vi "SigSyn-Set Property.vi"(0 "StimChan In":T1 caption="Stimulus" {"Filter"."Stages"."IIR Filter"."Forward Coefficients" format="%.4f"; "Filter"."Stages"."IIR Filter"."Reverse Coefficients" format="%.4f"}, 7 "Property":string, 9 "Value":dbl) -> (4 "StimChan Out":T1={"Waveform"={"Type"=enum."Tone", "Tone"={"Frequency (kHz)"=0.0, "Last Freq"=0.0, "Last Phase"=0.0}, "Pulse Train"={"Pulse width (us)"=0.0, "Pulse rate (Hz)"=0.0, "Gap (ms)"=0.0, "Polarity"=enum."POS", "PT State"={"Template"=[], "Nperiod"=0, "Index"=0, "Pulse Rate (Hz)"=0.0, "Phase (cycles)"=0.0, "Noff"=0}, "Asynch"=FALSE}, "Noise"={"InvFilt"=FALSE, "Noise"=[], "CurPt"=0, "Aweight"=FALSE, "Seed"=0, "afile"=path ""}, "File"={"Filename"=path "", "Signal"=[], "Channel"=0, "stream"=FALSE, "offset"=0, "nreps"=0, "loops"=0}, "FMSweep"={"Rate (oct/s)"=0.0, "Fmin (Hz)"=0.0, "Fmax (Hz)"=0.0, "Ramp (ms)"=0.0, "Linear"=FALSE}, "Chirp Train"={"Params"={"Fmin (kHz)"=4.0, "Fmax (kHz)"=64.0, "Compensate"=FALSE, "Duration (ms)"=2.0}, "Data"={"WF"=[]}}, "Complex Tone"={"Params"={"F0 (Hz)"=0.0, "Band"={"Flow (Hz)"=0.0, "Fhigh (Hz)"=0.0}, "Phase"=enum."Cosine", "Min F0 (Hz)"=0.0, "Max F0 (Hz)"=0.0, "ContinRandPhase"=FALSE, "Max peak factor"=inf, "Max mod depth"=2.0, "MinHarmNum"=0, "MaxHarmNum"=0, "Level Mode"=enum."per component", "% jitter"=0.0}, "Data"={"Ncomp"=0, "MinHarm"=0, "Phase"=[], "Amplitude"=[], "Npts/frame"=0, "Last F0"=0.0, "Fmin"=0.0, "Fmax"=0.0, "Lslope"=0.0, "randphase"=FALSE, "overall rms"=FALSE, "fmult"=[], "jittered"=FALSE}}, "Moving Ripple"={"Params"={"Fmin"=0.0, "Fmax"=0.0, "Density"=0.0, "Velocity"=0.0, "Depth"=0.0, "Phase"=0.0, "Comp/oct"=0}, "Data"={"Freq"=[], "A"=[], "phase"=[], "Phase"=0.0}}}, "Filter"={"Type"=enum."Lowpass", "CF (kHz)"=0.0, "BW (kHz)"=0.0, "Cascade"=FALSE, "Quadrature"=FALSE, "Scale Factor"=0.0, "Stages"=[], "Class"=enum."Elliptic", "Order"=0, "BWUnits"=enum."Linear"}, "Burst"={"Active"=FALSE, "Delay (ms)"=0.0, "Duration (ms)"=0.0, "Ramp (ms)"=0.0, "Rate (Hz)"=0.0, "Trepeat (ms)"=0.0, "Repeat"=FALSE}, "Level"={"Level"=0.0, "Units"=enum."dB atten", "Max"=0.0, "Multiplier"=0.0, "Cal File"=path "", "Cal"={"Freq (Hz)"=[], "Mag (dB SPL)"=[], "Phase (deg)"=[]}}, "Name"="", "Advanced"={"Rep Mask"="", "AltPol"=FALSE, "Var"="", "Expr"="", "Persist"=FALSE}, "SAM"={"Active"=FALSE, "Frequency (Hz)"=0.0, "Depth"=0.0, "Init Phase (cycles)"=0.0, "phase (degrees)"=0.0, "Asynch"=FALSE}} {"Filter"."Stages"."IIR Filter"."Forward Coefficients" format="%.4f"; "Filter"."Stages"."IIR Filter"."Reverse Coefficients" format="%.4f"})   [LabVIEW 2015]
uses:
  Controls/Stimulus Channel (Full)/Full Stimulus Channel Data.ctl
  Controls/Waveform XCtl/Waveform Data.ctl
  Controls/Waveform XCtl/Waveform Enum.ctl
  Waveform VIs/Tone VIs/Tone Params.ctl
  Waveform VIs/Pulse Train VIs/Pulse Train Params.ctl
  Waveform VIs/Pulse Train VIs/Pulse Polarity.ctl
  Waveform VIs/Pulse Train VIs/PT-Continuous State.ctl
  Waveform VIs/Noise VIs/Noise Params.ctl
  Waveform VIs/File VIs/StimFile-Params.ctl
  Waveform VIs/FM Sweep VIs/FM Sweep Params.ctl
  Waveform VIs/Chirp Train VIs/Chirp Train.ctl
  Waveform VIs/Chirp Train VIs/Chirp Train Params.ctl
  Waveform VIs/Complex Tone VIs/CT-Params.ctl
  Waveform VIs/Complex Tone VIs/CT-Phase Enum.ctl
  Waveform VIs/Complex Tone VIs/CT-Runtime Data.ctl
  Waveform VIs/Moving Ripple VIs/Moving Ripple.ctl
  Waveform VIs/Moving Ripple VIs/Moving Ripple.Params.ctl
  Waveform VIs/Moving Ripple VIs/Moving Ripple.Data.ctl
  Controls/Advanced Filter XCtl/Filter Data.ctl
  Filter VIs/Filter-Bandwidth Units.ctl
  Controls/Burst XCtl/Burst Data.ctl
  Controls/Level XCtl/Level Data.ctl
  Controls/Level XCtl/Level Units.ctl
  Controls/Advanced Options XCtl/Advanced Stimulus Options.ctl
  Modulation VIs/SAM VIs/SAM Params.ctl
  <vilib>/regexp/Match Regular Expression.xnode
  Controls/Advanced Filter XCtl/Advanced Filter XCtl.xctl
  Controls/Level XCtl/Level XCtl.xctl
  Controls/Burst XCtl/Burst Control.xctl
  Controls/Waveform XCtl/Waveform XCtl.xctl
  Controls/Advanced Options XCtl/Advanced Stimulus Options.xctl
  Controls/Stimulus Channel (Full)/Stimulus Channel (Full).xctl
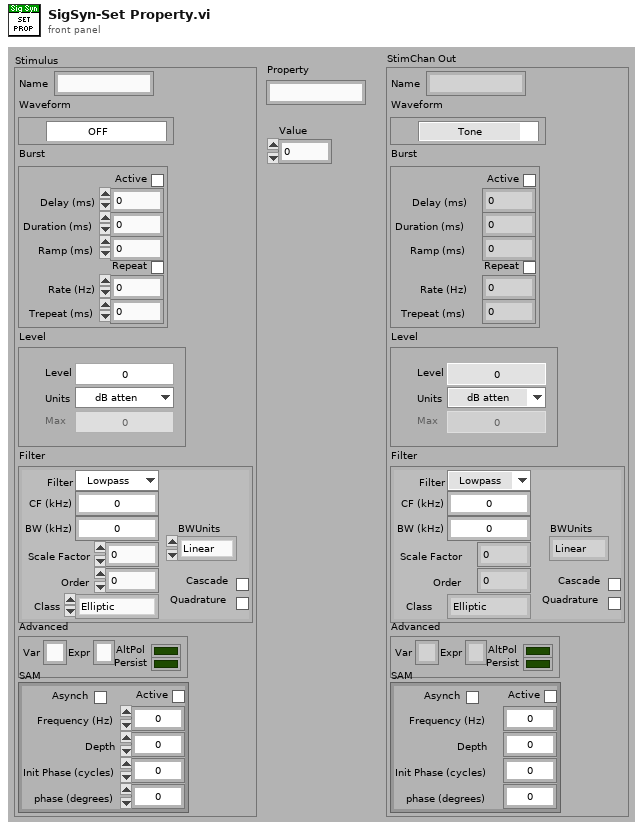
[diagram p1: front panel]
types:
  T1 = typedef "Stimulus Channel (Full).xctl/Full Stimulus Channel Data.ctl" = cluster{"Waveform":T2, "Filter":T19, "Burst":T21, "Level":T22, "Name":string, "Advanced":T24, "SAM":T25}
  T2 = typedef "Waveform XCtl.xctl/Waveform Data.ctl" = cluster{"Type":T3, "Tone":T4, "Pulse Train":T5, "Noise":T8, "File":T9, "FMSweep":T10, "Chirp Train":T11, "Complex Tone":cluster{"Params":T13, "Data":T15}, "Moving Ripple":T16}
  T3 = typedef "Waveform Enum.ctl" = enum16{"OFF", "Tone", "Noise", "Pulse Train", "File", "FM Sweep", "Chirp Train", "Complex Tone", "FM Tone", "Moving Ripple"}
  T4 = typedef "Tone Params.ctl" = cluster{"Frequency (kHz)":dbl, "Last Freq":dbl, "Last Phase":dbl}
  T5 = typedef "Pulse Train Params.ctl" = cluster{"Pulse width (us)":dbl, "Pulse rate (Hz)":dbl, "Gap (ms)":dbl, "Polarity":T6, "PT State":T7, "Asynch":bool}
  T6 = typedef "Pulse Polarity.ctl" = enum16{"POS", "NEG", "POS-NEG", "NEG-POS"}
  T7 = typedef "PT-Continuous State.ctl" = cluster{"Template":dbl[], "Nperiod":i32, "Index":i32, "Pulse Rate (Hz)":dbl, "Phase (cycles)":dbl, "Noff":i32}
  T8 = typedef "Noise Params.ctl" = cluster{"InvFilt":bool, "Noise":dbl[], "CurPt":i32, "Aweight":bool, "Seed":i32, "afile":path}
  T9 = typedef "StimFile-Params.ctl" = cluster{"Filename":path, "Signal":dbl[], "Channel":i32, "stream":bool, "offset":i32, "nreps":i32, "loops":i32}
  T10 = typedef "FM Sweep Params.ctl" = cluster{"Rate (oct/s)":dbl, "Fmin (Hz)":dbl, "Fmax (Hz)":dbl, "Ramp (ms)":dbl, "Linear":bool}
  T11 = typedef "Chirp Train.ctl" = cluster{"Params":T12, "Data":cluster{"WF":dbl[]}}
  T12 = typedef "Chirp Train Params.ctl" = cluster{"Fmin (kHz)":dbl, "Fmax (kHz)":dbl, "Compensate":bool, "Duration (ms)":dbl}
  T13 = typedef "CT-Params.ctl" = cluster{"F0 (Hz)":dbl, "Band":cluster{"Flow (Hz)":dbl, "Fhigh (Hz)":dbl}, "Phase":T14, "Min F0 (Hz)":dbl, "Max F0 (Hz)":dbl, "ContinRandPhase":bool, "Max peak factor":dbl, "Max mod depth":dbl, "MinHarmNum":i32, "MaxHarmNum":i32, "Level Mode":enum16{"per component", "overall rms"}, "% jitter":dbl}
  T14 = typedef "CT-Phase Enum.ctl" = enum16{"Cosine", "Random", "Alternating"}
  T15 = typedef "CT-Runtime Data.ctl" = cluster{"Ncomp":i32, "MinHarm":i32, "Phase":dbl[], "Amplitude":dbl[], "Npts/frame":i32, "Last F0":dbl, "Fmin":dbl, "Fmax":dbl, "Lslope":dbl, "randphase":bool, "overall rms":bool, "fmult":dbl[], "jittered":bool}
  T16 = typedef "Moving Ripple.ctl" = cluster{"Params":T17, "Data":T18}
  T17 = typedef "Moving Ripple.Params.ctl" = cluster{"Fmin":dbl, "Fmax":dbl, "Density":dbl, "Velocity":dbl, "Depth":dbl, "Phase":dbl, "Comp/oct":i32}
  T18 = typedef "Moving Ripple.Data.ctl" = cluster{"Freq":dbl[], "A":dbl[], "phase":dbl[], "Phase":dbl}
  T19 = typedef "Advanced Filter XCtl.xctl/Filter Data.ctl" = cluster{"Type":enum16{"Lowpass", "Highpass", "Bandpass", "Bandstop", "OFF"}, "CF (kHz)":dbl, "BW (kHz)":dbl, "Cascade":bool, "Quadrature":bool, "Scale Factor":dbl, "Stages":cluster{"IIR Filter":cluster{"filter structure":enum32{"IIR 2nd Order", "IIR 4th Order"}, "Reverse Coefficients":dbl[], "Forward Coefficients":dbl[]}, "State":dbl[]}[], "Class":enum16{"Elliptic", "Butterworth"}, "Order":i32, "BWUnits":T20}
  T20 = typedef "Filter-Bandwidth Units.ctl" = enum16{"Linear", "Octaves", "Min-Max"}
  T21 = typedef "Burst Control.xctl/Burst Data.ctl" = cluster{"Active":bool, "Delay (ms)":dbl, "Duration (ms)":dbl, "Ramp (ms)":dbl, "Rate (Hz)":dbl, "Trepeat (ms)":dbl, "Repeat":bool}
  T22 = typedef "Level XCtl.xctl/Level Data.ctl" = cluster{"Level":dbl, "Units":T23, "Max":dbl, "Multiplier":dbl, "Cal File":path, "Cal":cluster{"Freq (Hz)":dbl[], "Mag (dB SPL)":dbl[], "Phase (deg)":dbl[]}}
  T23 = typedef "Level Units.ctl" = enum16{"dB atten", "dB SPL", "dB re 1 Vrms", "dB V/Hz½", "mW", "dB HL", "Volts", "dB mW"}
  T24 = typedef "Advanced Stimulus Options.xctl/Advanced Stimulus Options.ctl" = cluster{"Rep Mask":string, "AltPol":bool, "Var":string, "Expr":string, "Persist":bool}
  T25 = typedef "SAM Params.ctl" = cluster{"Active":bool, "Frequency (Hz)":dbl, "Depth":dbl, "Init Phase (cycles)":dbl, "phase (degrees)":dbl, "Asynch":bool}
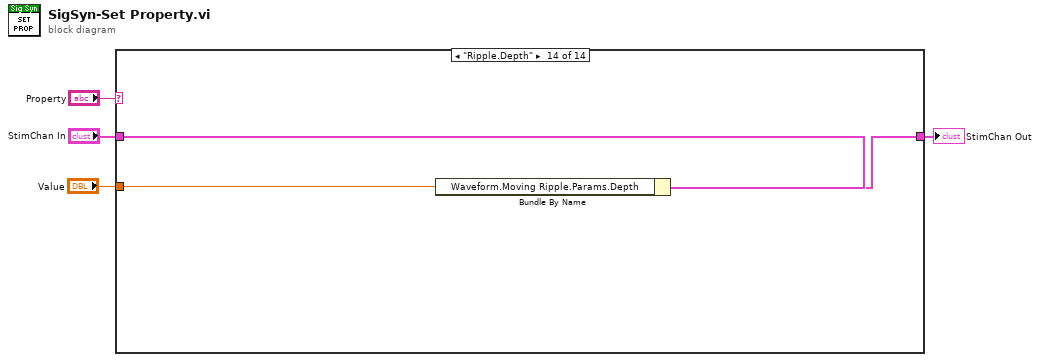
[diagram p0: block diagram]
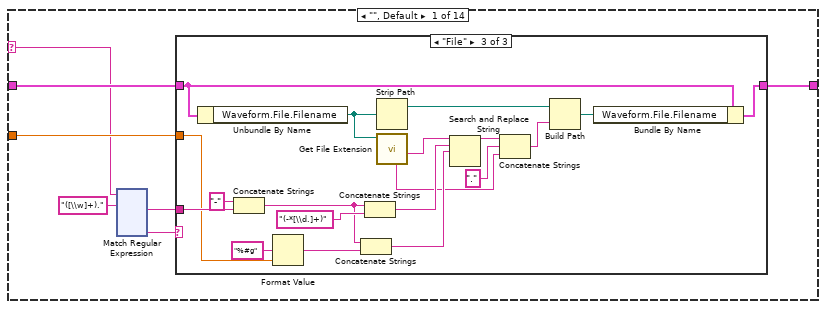
[diagram p2: hidden frame]
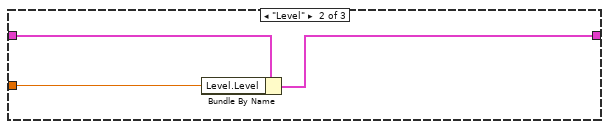
[diagram p4: hidden frame]
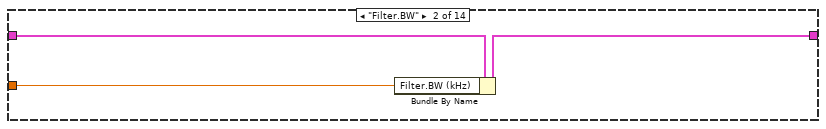
[diagram p5: hidden frame]
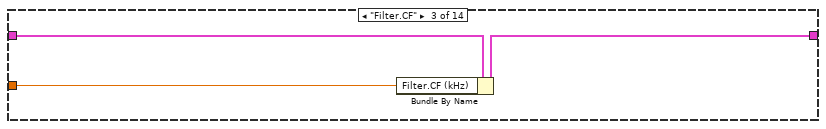
[diagram p6: hidden frame]
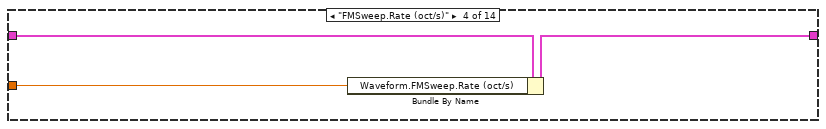
[diagram p7: hidden frame]
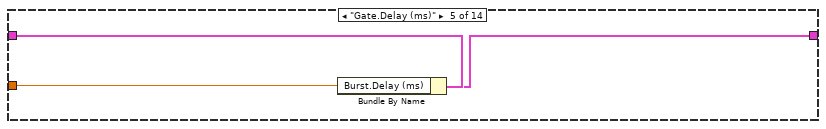
[diagram p8: hidden frame]
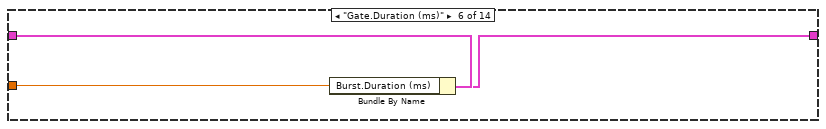
[diagram p9: hidden frame]
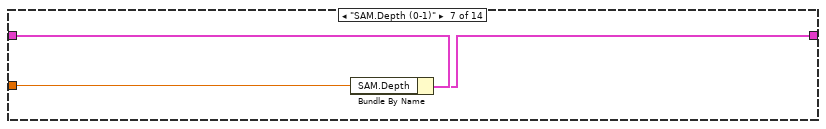
[diagram p10: hidden frame]
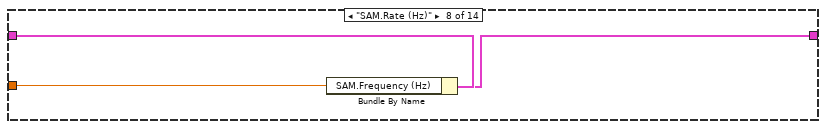
[diagram p11: hidden frame]
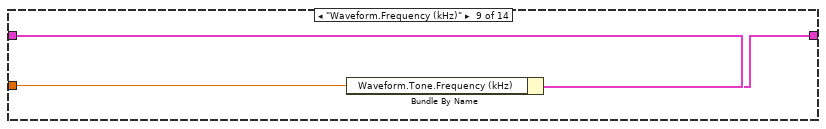
[diagram p12: hidden frame]
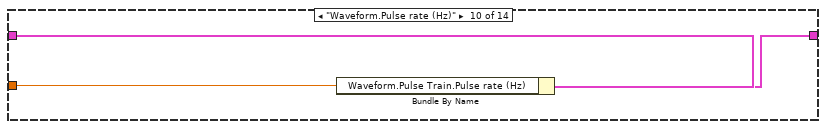
[diagram p13: hidden frame]
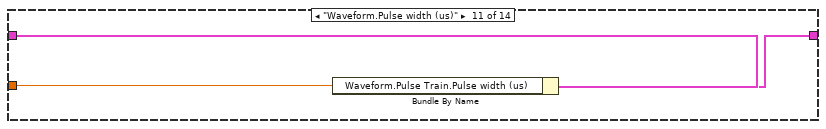
[diagram p14: hidden frame]
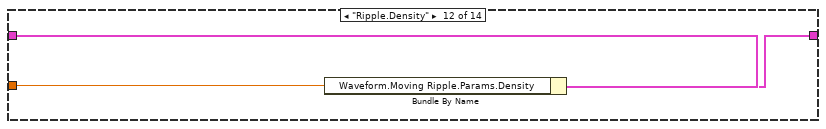
[diagram p15: hidden frame]
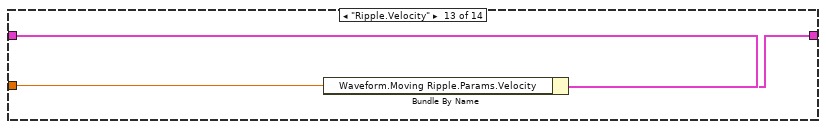
[diagram p16: hidden frame]
diagram:
  n1 = case shown="\"Ripple.Depth\"" "Property" {
    selector: "Property" -> [w7 _ _ _ _ _ _ _ _ _ _ _ _ _]
    tunnel: "StimChan In" -> [w11 w153 w156 w159 w162 w165 w168 w171 w174 w177 w180 w183 w186 w189]
    tunnel: [w10 w152 w155 w158 w161 w164 w167 w170 w173 w176 w179 w182 w185 w188] -> w2
    tunnel: "Value" -> [w9 w151 w154 w157 w160 w163 w166 w169 w172 w175 w178 w181 w184 w187]
    frame "", Default {
      n2 = xnode "Match Regular Expression"("input string"=w7, "regular expression"="([\\w]+).") -> ("after match"=w5:string, "submatch 1"=w6:string)  [unwired: 4 in, 4 out]
      n3 = case shown="\"File\"" w6 {
        tunnel: w11 -> [w128 w131 w150]
        tunnel: [w128 w130 w144] -> w10
        tunnel: w9 -> [_ w129 w147]
        tunnel: w5 -> [_ _ w149]
        frame "", Default {
        }
        frame "Level" {
          n4 = Bundle By Name(cluster=w131, "Level.Level"=w129) -> (w130:T1)
        }
        frame "File" {
          n5 = Unbundle By Name(w150) -> ("Waveform.File.Filename"=w138:path)
          n6 = Concatenate Strings("-" ("string"), w149) -> (w140:string)
          n7 = Format Value(format string="%#g", value (0)=w147) -> (output string=w145:string)  [unwired: 1 in]
          n8 = Concatenate Strings(w140, w145) -> (w141:string)
          n9 = Concatenate Strings(w140, "(-*[\\d.]+)" ("string")) -> (w143:string)
          n10 = Strip Path(path=w138) -> (stripped path=w137:path)  [unwired: 1 out]
          n11 = call <vilib>:"Get File Extension.vi"("file"=w138) -> ("filename without extension"=w139:string, "unmodified file extension"=w133:string)  [unwired: 6 in, 3 out]
          n12 = Search and Replace String(input string=w139, search string=w143, replace string=w141) -> (result string=w135:string)  [unwired: 5 in, 3 out]
          n13 = Concatenate Strings(w135, "." ("string"), w133) -> (w134:string)
          n14 = Build Path(base path=w137, name or relative path=w134) -> (appended path=w136:path)
          n15 = Bundle By Name(cluster=w150, "Waveform.File.Filename"=w136) -> (w144:T1)
        }
      }
    }
    frame "Filter.BW" {
      n16 = Bundle By Name(cluster=w153, "Filter.BW (kHz)"=w151) -> (w152:T1)
    }
    frame "Filter.CF" {
      n17 = Bundle By Name(cluster=w156, "Filter.CF (kHz)"=w154) -> (w155:T1)
    }
    frame "FMSweep.Rate (oct/s)" {
      n18 = Bundle By Name(cluster=w159, "Waveform.FMSweep.Rate (oct/s)"=w157) -> (w158:T1)
    }
    frame "Gate.Delay (ms)" {
      n19 = Bundle By Name(cluster=w162, "Burst.Delay (ms)"=w160) -> (w161:T1)
    }
    frame "Gate.Duration (ms)" {
      n20 = Bundle By Name(cluster=w165, "Burst.Duration (ms)"=w163) -> (w164:T1)
    }
    frame "SAM.Depth (0-1)" {
      n21 = Bundle By Name(cluster=w168, "SAM.Depth"=w166) -> (w167:T1)
    }
    frame "SAM.Rate (Hz)" {
      n22 = Bundle By Name(cluster=w171, "SAM.Frequency (Hz)"=w169) -> (w170:T1)
    }
    frame "Waveform.Frequency (kHz)" {
      n23 = Bundle By Name(cluster=w174, "Waveform.Tone.Frequency (kHz)"=w172) -> (w173:T1)
    }
    frame "Waveform.Pulse rate (Hz)" {
      n24 = Bundle By Name(cluster=w177, "Waveform.Pulse Train.Pulse rate (Hz)"=w175) -> (w176:T1)
    }
    frame "Waveform.Pulse width (us)" {
      n25 = Bundle By Name(cluster=w180, "Waveform.Pulse Train.Pulse width (us)"=w178) -> (w179:T1)
    }
    frame "Ripple.Density" {
      n26 = Bundle By Name(cluster=w183, "Waveform.Moving Ripple.Params.Density"=w181) -> (w182:T1)
    }
    frame "Ripple.Velocity" {
      n27 = Bundle By Name(cluster=w186, "Waveform.Moving Ripple.Params.Velocity"=w184) -> (w185:T1)
    }
    frame "Ripple.Depth" {
      n28 = Bundle By Name(cluster=w189, "Waveform.Moving Ripple.Params.Depth"=w187) -> (w188:T1)
    }
  }
  "StimChan Out" <- w2
